vi "BRig_Host__Loop_Producer__UploadClosedLoop__v3.vi"(0 "session handle":T1, 1 "input_webdav_status":bool, 4 "testNewLaserSettings":bool, 5 "input_array":u16[](array[numeric]), 6 "input_arrayBuffer":u16[][](array[numeric]), 8 "input_arrayBuffer_length":i32) -> (10 "output_arrayBuffer_length":i32, 12 "output_arrayBuffer":u16[][](array[numeric]))   [LabVIEW 2014]
uses:
  <vilib>/WebDAVClient/Advanced/SessionHandle.ctl
  <vilib>/Utility/file.llb/Write To Spreadsheet File (I64).vi
  <vilib>/WebDAVClient/Advanced/Put File.vi
  <vilib>/WebDAVClient/NI_WebDAV.lvlib
panel:
  out "Sent":bool
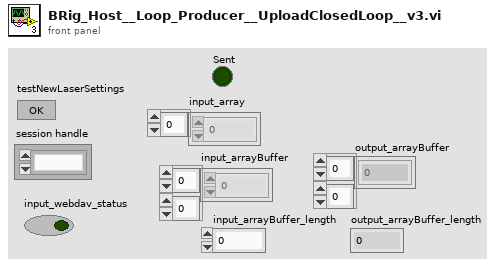
[diagram p1: front panel]
types:
  T1 = typedef "NI_WebDAV.lvlib/SessionHandle.ctl" = refnum<k1>
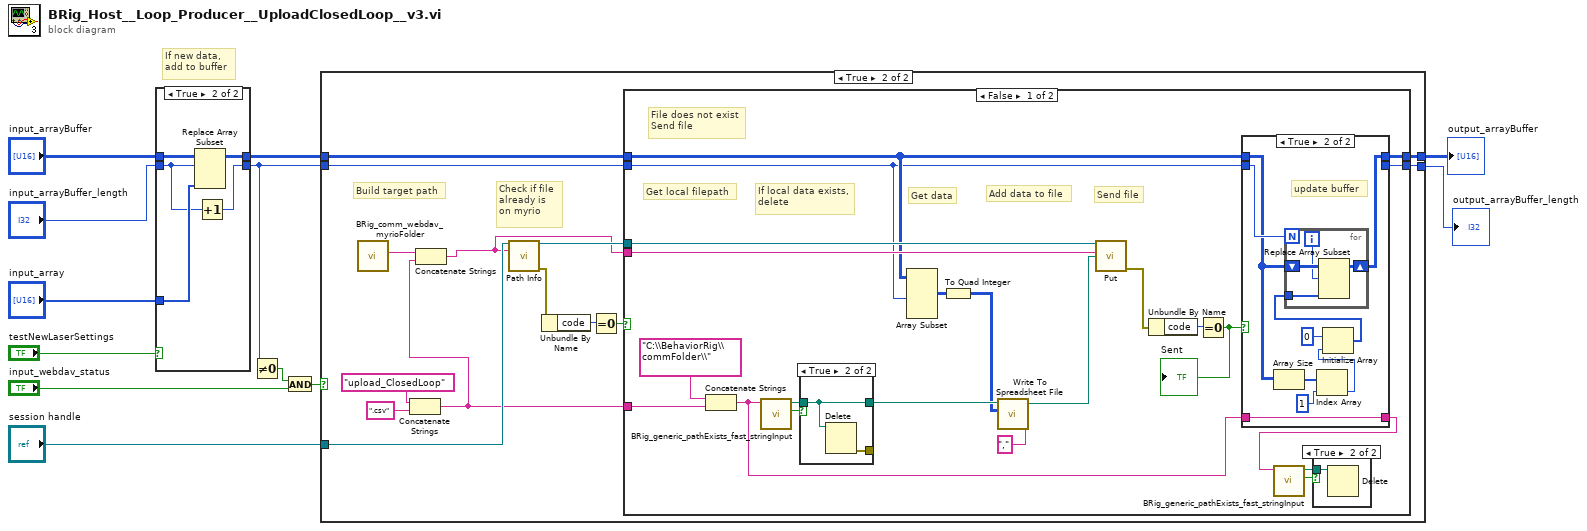
[diagram p0: block diagram]
diagram:
  # "If new data,\nadd to buffer"
  n1 = case shown="True" "testNewLaserSettings" {
    tunnel: "input_arrayBuffer" -> [w14 w19]
    tunnel: [w14 w17] -> w7
    tunnel: [w13 w15] -> w4
    tunnel: "input_arrayBuffer_length" -> [w13 w16]
    tunnel: "input_array" -> [_ w18]
    frame False {
    }
    frame True {
      n2 = Replace Array Subset(array=w19, new element=w18, index (row)=w16) -> (w17:u16[][])  [unwired: 1 in]
      n3 = Increment(x=w16) -> (x+1=w15:i32)
    }
  }
  n4 = Not Equal To 0?(x=w4) -> (x != 0?=w2:bool)
  n5 = And(x=w2, y="input_webdav_status") -> (x .and. y?=w1:bool)
  n6 = case shown="True" w1 {
    tunnel: "session handle" -> [_ w30]
    tunnel: w7 -> [w21 w28]
    tunnel: [w21 w27] -> w11
    tunnel: w4 -> [w20 w26]
    tunnel: [w20 w25] -> w10
    frame False {
    }
    frame True {
      # "Check if file\nalready is\non myrio"
      # "Build target path"
      n7 = call "BRig_comm_webdav_myrioFolder.vi"() -> ("output_myrioFolder"=w33:string)  [unwired: 11 in]
      n8 = Concatenate Strings("upload_ClosedLoop" ("string"), ".csv" ("string")) -> (w24:string)
      n9 = Concatenate Strings(w33, w24) -> (w22:string)
      n10 = call <vilib>:"Path Info.vi"("session handle"=w30, "relative uri"=w22) -> ("session handle out"=w23:T1, "error out"=w31:errorcluster)  [unwired: 10 in, 2 out]
      n11 = Unbundle By Name(w31) -> ("code"=w32:i32)
      n12 = Equal To 0?(x=w32) -> (x = 0?=w29:bool)
      n13 = case shown="False" w29 {
        tunnel: w28 -> [w44 w79]
        tunnel: [w43 w79] -> w27
        tunnel: w26 -> [w42 w78]
        tunnel: [w41 w78] -> w25
        tunnel: w24 -> [w56 _]
        tunnel: w23 -> [w47 _]
        tunnel: w22 -> [w46 _]
        frame False {
          # "Send file"
          # "Add data to file"
          # "Get data"
          # "If local data exists,\ndelete"
          # "Get local filepath"
          # "File does not exist\nSend file"
          n14 = Concatenate Strings("C:\\BehaviorRig\\commFolder\\", w56) -> (w37:string)
          n15 = call "BRig_generic_pathExists_fast_stringInput.vi"("input_filePath"=w37) -> ("output_Iexist"=w55:bool, "output_filePath"=w54:path)  [unwired: 8 in, 1 out]
          n16 = case shown="True" w55 {
            tunnel: w54 -> [w75 w76]
            tunnel: [_ w77] -> _
            tunnel: [w75 w76] -> w51
            frame False {
            }
            frame True {
              n17 = Delete(path (use dialog)=w76) -> (error out=w77:errorcluster)  [unwired: 4 in, 2 out]
            }
          }
          n18 = Array Subset(array=w44, length (row)=w42) -> (w53:u16[][])  [unwired: 3 in]
          n19 = To Quad Integer(1:w53) -> (0:w50:i64[][])
          n20 = call-poly <vilib>:"Write To Spreadsheet File.vi"("delimiter (\\t)"="," ("delimiter (\\t)"), "2D data"=w50, "file path (dialog if empty)"=w51) -> ("new file path (Not A Path if cancelled)"=w40:path)  [unwired: 5 in]
          n21 = call-poly <vilib>:"Put.vi"("session handle"=w47, "relative uri"=w46, "local file path"=w40) -> ("error out"=w49:errorcluster)  [unwired: 10 in, 2 out]
          n22 = Unbundle By Name(w49) -> ("code"=w48:i32)
          n23 = Equal To 0?(x=w48) -> (x = 0?=w45:bool)
          "Sent" <- w45
          n24 = case shown="True" w45 {
            tunnel: w44 -> [w61 w65]
            tunnel: [w61 w63] -> w43
            tunnel: w42 -> [w60 w70]
            tunnel: [w60 _] -> w41
            tunnel: w37 -> [w59 w62]
            tunnel: [w59 w62] -> w36
            frame False {
            }
            frame True {
              # "update buffer"
              n25 = Array Size(array=w65) -> (size(s)=w69:i32[])
              n26 = Index Array(array=w69, index=1) -> (element=w67:i32)
              n27 = Initialize Array(u16 0 ("element"), w67) -> (w64:u16[])
              n28 = for {
                N: w70 -> [_]
                shift-right: [w73] -> w63
                shift-left: w65 -> [w74]
                tunnel: w64 -> [w71]
                i -> [w72]
                n29 = Replace Array Subset(array=w74, new element=w71, index (row)=w72) -> (w73:u16[][])  [unwired: 1 in]
              }
            }
          }
          n30 = call "BRig_generic_pathExists_fast_stringInput.vi"("input_filePath"=w36) -> ("output_Iexist"=w38:bool, "output_filePath"=w39:path)  [unwired: 8 in, 1 out]
          n31 = case shown="True" w38 {
            tunnel: w39 -> [_ w58]
            frame False {
            }
            frame True {
              n32 = Delete(path (use dialog)=w58) -> ()  [unwired: 4 in, 3 out]
            }
          }
        }
        frame True {
          # "File does exist\nWait for myrio to process it"
        }
      }
    }
  }
  "output_arrayBuffer" <- w11
  "output_arrayBuffer_length" <- w10
